vi "sr400_software_trigger.vi"(8 "error in (no error)":errorcluster, 10 "Settings In":T2={"Channel A"={"Input"=0, "A Discriminator Level (V)"=0.0, "A Discriminator Slope"=enum."Falling", "A Gate Mode"=enum."CW", "A Gate Delay (s)"=0.0, "A Gate Width (s)"=5e-09, "Scan Increment (s)"=0.0}, "Channel B"={"Input"=0, "B Discriminator Level (V)"=0.0, "B Discriminator Slope"=enum."Falling", "B Gate Mode"=enum."CW", "B Gate Delay (s)"=0.0, "B Gate Width (s)"=5e-09, "Scan Increment (s)"=0.0}, "Channel T"={"Input"=0, "Trigger Level (V)"=0.0, "Trigger Slope"=enum."Falling", "T Discriminator Slope"=enum."Falling", "T Discriminator Level (V)"=0.0, "Trigger Preset"=1.0}, "N Periods"=0.0, "At N"=enum."Stop", "Counting Mode"=enum."A,B for T Preset", "GPIB Address"="", "Dwell Time (s)"=0.002, "Port 1 Mode"=0, "Port 1 Voltage"=0.0, "Port 1 Scan Increment"=-0.5, "Port 2 Voltage"=0.0, "Port 2 Scan Increment"=0.0, "Port 2 Mode"=0, "Counter Toggle"=FALSE, "Pusleblater Settings"={"Loop Start Channel"=0.0, "Loop End Channel"=0.0, "Loop On"=FALSE}} {"Port 2 Mode" items=["Scan"=1, "Fixed"=0]; "Port 2 Scan Increment" min=-0.5 max=0.5; "Port 2 Voltage" min=-10.0 max=10.0; "Port 1 Scan Increment" min=-0.5 max=-0.5; "Port 1 Voltage" min=-10.0 max=10.0; "Port 1 Mode" items=["Scan"=1, "Fixed"=0]; "Dwell Time (s)" min=0.002 max=60.0 format="%#_6p"; "N Periods" min=0.0 max=2000.0 step=1.0; "Channel T"."Trigger Preset" min=1.0 max=900000000000.0 format="%#_1e"; "Channel T"."T Discriminator Level (V)" min=-0.3 max=0.3 format="%#_6p"; "Channel T"."Trigger Level (V)" min=-2.0 max=2.0 format="%#_6p"; "Channel T"."Input" items=["10 MHz", "Input 2", "Trig"]; "Channel B"."Scan Increment (s)" min=0.0 max=0.09992 format="%#_6p"; "Channel B"."B Gate Width (s)" min=5e-09 max=0.9992 format="%#_6p"; "Channel B"."B Gate Delay (s)" min=0.0 max=0.9992 format="%#_6p"; "Channel B"."B Discriminator Level (V)" min=-0.3 max=0.3 format="%#_6p"; "Channel B"."Input" items=["Input 2"=2, "Input 1"=1]; "Channel A"."Scan Increment (s)" min=0.0 max=0.09992 format="%#_6p"; "Channel A"."A Gate Width (s)" min=5e-09 max=0.9992 format="%#_6p"; "Channel A"."A Gate Delay (s)" min=0.0 max=0.9992 format="%#_6p"; "Channel A"."A Discriminator Level (V)" min=-0.3 max=0.3 format="%#_6p"; "Channel A"."Input" items=["Input 1", "10 MHz"]}) -> (0 "error out":errorcluster, 2 "Settings Out":T2={"Channel A"={"Input"=0, "A Discriminator Level (V)"=0.0, "A Discriminator Slope"=enum."Falling", "A Gate Mode"=enum."CW", "A Gate Delay (s)"=0.0, "A Gate Width (s)"=5e-09, "Scan Increment (s)"=0.0}, "Channel B"={"Input"=0, "B Discriminator Level (V)"=0.0, "B Discriminator Slope"=enum."Falling", "B Gate Mode"=enum."CW", "B Gate Delay (s)"=0.0, "B Gate Width (s)"=5e-09, "Scan Increment (s)"=0.0}, "Channel T"={"Input"=0, "Trigger Level (V)"=0.0, "Trigger Slope"=enum."Falling", "T Discriminator Slope"=enum."Falling", "T Discriminator Level (V)"=0.0, "Trigger Preset"=1.0}, "N Periods"=0.0, "At N"=enum."Stop", "Counting Mode"=enum."A,B for T Preset", "GPIB Address"="", "Dwell Time (s)"=0.002, "Port 1 Mode"=0, "Port 1 Voltage"=0.0, "Port 1 Scan Increment"=-0.5, "Port 2 Voltage"=0.0, "Port 2 Scan Increment"=0.0, "Port 2 Mode"=0, "Counter Toggle"=FALSE, "Pusleblater Settings"={"Loop Start Channel"=0.0, "Loop End Channel"=0.0, "Loop On"=FALSE}} {"Port 2 Mode" items=["Scan"=1, "Fixed"=0]; "Port 2 Scan Increment" min=-0.5 max=0.5; "Port 2 Voltage" min=-10.0 max=10.0; "Port 1 Scan Increment" min=-0.5 max=-0.5; "Port 1 Voltage" min=-10.0 max=10.0; "Port 1 Mode" items=["Scan"=1, "Fixed"=0]; "Dwell Time (s)" min=0.002 max=60.0 format="%#_6p"; "N Periods" min=0.0 max=2000.0 step=1.0; "Channel T"."Trigger Preset" min=1.0 max=900000000000.0 format="%#_1e"; "Channel T"."T Discriminator Level (V)" min=-0.3 max=0.3 format="%#_6p"; "Channel T"."Trigger Level (V)" min=-2.0 max=2.0 format="%#_6p"; "Channel T"."Input" items=["10 MHz", "Input 2", "Trig"]; "Channel B"."Scan Increment (s)" min=0.0 max=0.09992 format="%#_6p"; "Channel B"."B Gate Width (s)" min=5e-09 max=0.9992 format="%#_6p"; "Channel B"."B Gate Delay (s)" min=0.0 max=0.9992 format="%#_6p"; "Channel B"."B Discriminator Level (V)" min=-0.3 max=0.3 format="%#_6p"; "Channel B"."Input" items=["Input 2"=2, "Input 1"=1]; "Channel A"."Scan Increment (s)" min=0.0 max=0.09992 format="%#_6p"; "Channel A"."A Gate Width (s)" min=5e-09 max=0.9992 format="%#_6p"; "Channel A"."A Gate Delay (s)" min=0.0 max=0.9992 format="%#_6p"; "Channel A"."A Discriminator Level (V)" min=-0.3 max=0.3 format="%#_6p"; "Channel A"."Input" items=["Input 1", "10 MHz"]})   [LabVIEW 2013]
uses:
  Controls/SR400/SR400.ctl
  Controls/SR400/Channel A/channelA.ctl
  Controls/SR400/Channel A/channelA_inputs.ctl
  Controls/SR400/discrim_slope.ctl
  Controls/SR400/gate_mode.ctl
  Controls/SR400/Channel B/channelB.ctl
  Controls/SR400/Channel B/inputsB.ctl
  Controls/SR400/Channel T/channelT.ctl
  Controls/SR400/Channel T/inputsT.ctl
  <vilib>/Instr/_visa.llb/GPIB Status Boolean Array.ctl
panel:
  out "ibsta":T1
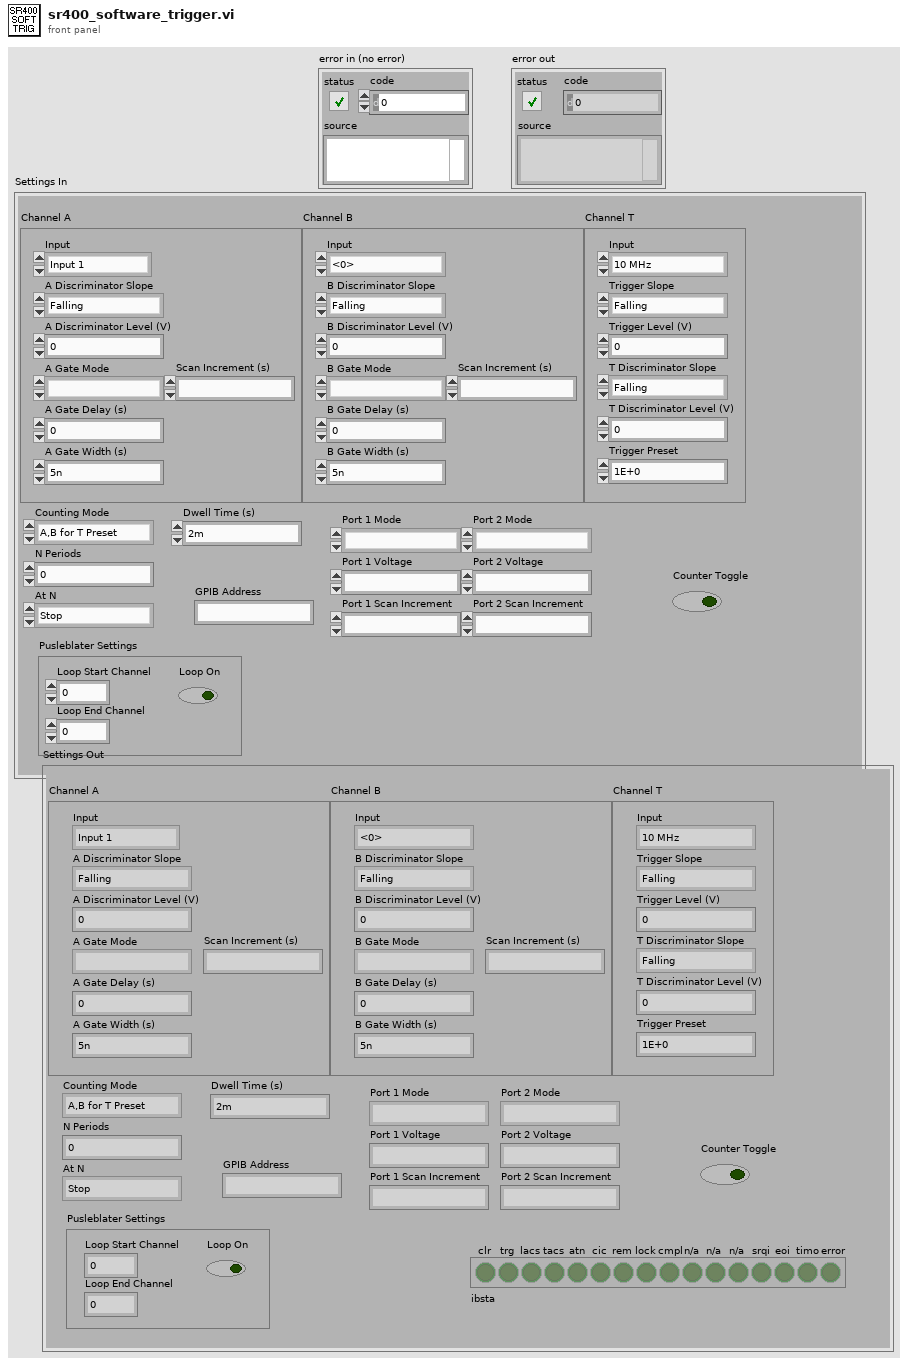
[diagram p1: front panel]
types:
  T1 = typedef "GPIB Status Boolean Array.ctl" = bool[]
  T2 = typedef "SR400.ctl" = cluster{"Channel A":T3, "Channel B":T7, "Channel T":T9, "N Periods":dbl, "At N":enum16{"Stop", "Start"}, "Counting Mode":enum16{"A,B for T Preset", "A-B for T Preset", "A+B for T Preset"}, "GPIB Address":string, "Dwell Time (s)":dbl, "Port 1 Mode":i32, "Port 1 Voltage":dbl, "Port 1 Scan Increment":dbl, "Port 2 Voltage":dbl, "Port 2 Scan Increment":dbl, "Port 2 Mode":i32, "Counter Toggle":bool, "Pusleblater Settings":cluster{"Loop Start Channel":dbl, "Loop End Channel":dbl, "Loop On":bool}}
  T3 = typedef "channelA.ctl" = cluster{"Input":T4, "A Discriminator Level (V)":dbl, "A Discriminator Slope":T5, "A Gate Mode":T6, "A Gate Delay (s)":dbl, "A Gate Width (s)":dbl, "Scan Increment (s)":dbl}
  T4 = typedef "channelA_inputs.ctl" = u16
  T5 = typedef "discrim_slope.ctl" = enum16{"Rising", "Falling"}
  T6 = typedef "gate_mode.ctl" = enum16{"CW", "Fixed", "Scan"}
  T7 = typedef "channelB.ctl" = cluster{"Input":T8, "B Discriminator Level (V)":dbl, "B Discriminator Slope":T5, "B Gate Mode":T6, "B Gate Delay (s)":dbl, "B Gate Width (s)":dbl, "Scan Increment (s)":dbl}
  T8 = typedef "inputsB.ctl" = u16
  T9 = typedef "channelT.ctl" = cluster{"Input":T10, "Trigger Level (V)":dbl, "Trigger Slope":T5, "T Discriminator Slope":T5, "T Discriminator Level (V)":dbl, "Trigger Preset":dbl}
  T10 = typedef "inputsT.ctl" = u16
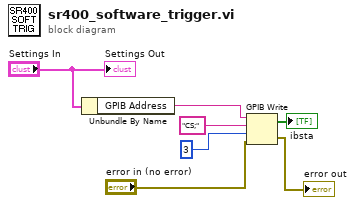
[diagram p0: block diagram]
diagram:
  n1 = Unbundle By Name("Settings In") -> ("GPIB Address"=w6:string)
  n2 = GPIB Write(0:w6, 1:"CS;" ("data"), 2:i16 3 ("mode (0)"), 3:"error in (no error)") -> (5:→"ibsta":bool[], 6:→"error out":errorcluster)  [unwired: 1 in]
  "Settings Out" <- "Settings In"
